vi "mes~产品出站.vi"(8 "error in (no error)":errorcluster caption="错误输入（无错误）", 11 "测试结果":string caption="测试结果:") -> (0 "error out":errorcluster caption="错误输出", 2 "出站成功":bool)   [LabVIEW 2015]
uses:
  ctl/SendOutStationCommon.ctl
  ctl/ReceiveOutStationCommon.ctl
  Global.vi
panel:
  in  "Headers":string[][](array[string])=[["Content-Type", "text/xml;charset=UTF-8"], ["SOAPAction", "\"http://tempuri.org/IOutStationServiceImpl/outStationService\""], ["Connection", "Keep-Alive"], ["User-Agent", "Apache-HttpClient/4.1.1 (java 1.5)"]]
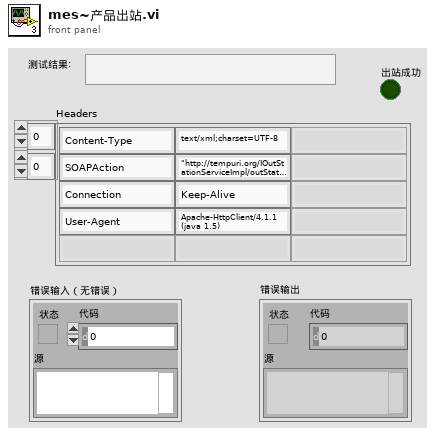
[diagram p1: front panel]
types:
  T1 = typedef "SendOutStationCommon.ctl" = cluster{"#attributes":cluster{"xmlns:soapenv":string, "xmlns:tem":string, "xmlns:cal":string}, "soapenv:Header":string, "soapenv:Body":cluster{"tem:outStationService":cluster{"tem:model":cluster{"cal:completeQty":string, "cal:equipNum":string, "cal:identiftyList":cluster{"cal:OutStationV01":cluster{"cal:identification":string, "cal:qualityStatus":string}[]}, "cal:productType":string, "cal:siteCode":string, "cal:testOrderNum":string}}}}
  T2 = cluster{"接口地址(URL)":string, "设备编号(equipNum)":string, "站点名称(siteCode)":string, "生产类型(productType)":string, "试验单号(testOrderNum)":string}
  T3 = typedef "ReceiveOutStationCommon.ctl" = cluster{"#attributes":cluster{"xmlns:s":string}, "s:Body":cluster{"outStationServiceResponse":cluster{"#attributes":cluster{"xmlns":string}, "outStationServiceResult":cluster{"#attributes":cluster{"xmlns:a":string, "xmlns:i":string}, "a:ErrorCode":string, "a:ErrorMessage":string, "a:Success":string}}}}
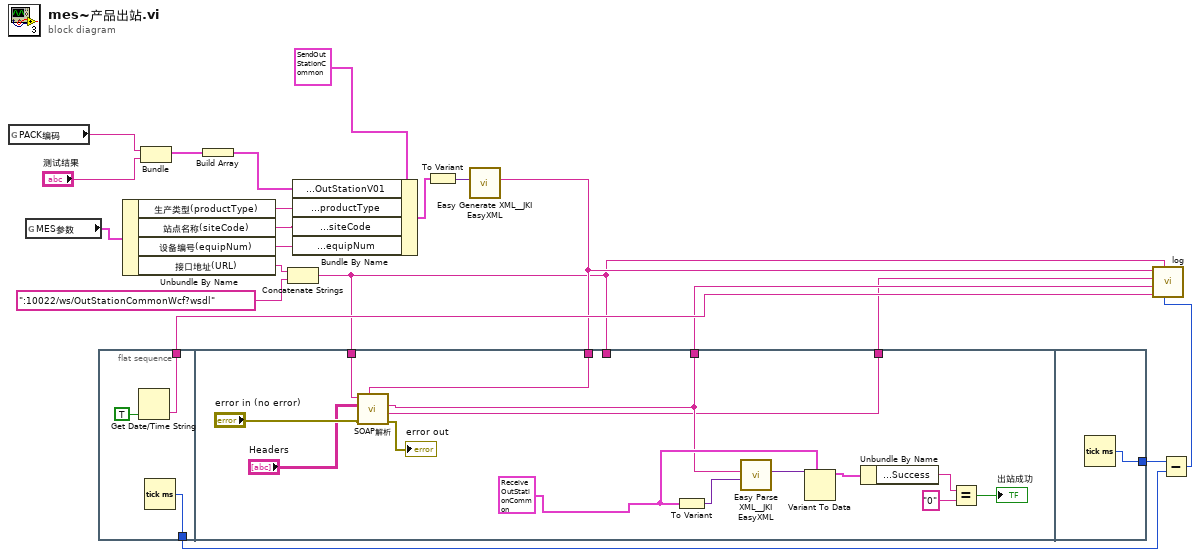
[diagram p0: block diagram]
diagram:
  n1 = global read "Global.vi" "PACK编码"() -> (w13:string)
  n2 = global read "Global.vi" "MES参数"() -> (w17:T2)
  n3 = flat-sequence {
    tunnel: [w23] -> w8
    tunnel: [w22] -> w7
    tunnel: w2 -> [_]
    tunnel: w5 -> [w28]
    tunnel: [w27] -> w4
    tunnel: w2 -> [w29]
    tunnel: [w25] -> w1
    tunnel: [w39] -> w9
    frame #0 {
      n4 = Get Date/Time String(want seconds? (F)=TRUE ("需要秒？(F)")) -> (time string=w22:string)  [unwired: 2 in, 1 out]
      n5 = Tick Count (ms)() -> (millisecond timer value=w23:u32)
    }
    frame #1 {
      w32 = T3 {"#attributes"={"xmlns:s"="http://schemas.xmlsoap.org/soap/envelope/"}, "s:Body"={"outStationServiceResponse"={"#attributes"={"xmlns"="http://tempuri.org/"}, "outStationServiceResult"={"#attributes"={"xmlns:a"="http://schemas.datacontract.org/2004/07/EdgeUtility", "xmlns:i"="http://www.w3.org/2001/XMLSchema-instance"}, "a:ErrorCode"="", "a:ErrorMessage"="", "a:Success"=""}}}} ("s:Envelope")
      n6 = call "SOAP解析.vi"("DATA"=w28, "错误输入（无错误）"="error in (no error)", "Headers"="Headers", "URL"=w29) -> ("错误输出"=→"error out":errorcluster, "headers"=w25:string, "body"=w27:string)  [unwired: 5 in]
      n7 = To Variant(anything=w32) -> (Variant=w38:variant)
      n8 = call <vilib>:"Easy Parse XML__JKI EasyXML.vi"("LabVIEW Data (Type)"=w38, "XML String"=w27) -> ("LabVIEW Data"=w37:variant)  [unwired: 8 in, 1 out]
      n9 = Variant To Data(type=w32, Variant=w37) -> (data=w36:T3)  [unwired: 1 in, 1 out]
      n10 = Unbundle By Name(w36) -> ("s:Body.outStationServiceResponse.outStationServiceResult.a:Success"=w35:string)
      n11 = Equal?(x=w35, y="0") -> (x = y?=→"出站成功":bool)
    }
    frame #2 {
      n12 = Tick Count (ms)() -> (millisecond timer value=w39:u32)
    }
  }
  n13 = Unbundle By Name(w17) -> ("生产类型(productType)"=w14:string, "站点名称(siteCode)"=w18:string, "设备编号(equipNum)"=w19:string, "接口地址(URL)"=w16:string)
  n14 = Bundle("PACK编码"=w13, "测试结果"="测试结果") -> (w11:cluster{"PACK编码":string, "测试结果":string})  [unwired: 1 in]
  n15 = Build Array(w11) -> (w10:cluster{"PACK编码":string, "测试结果":string}[])
  n16 = Concatenate Strings(w16, ":10022/ws/OutStationCommonWcf?wsdl") -> (w2:string)
  n17 = Bundle By Name(cluster=T1 {"#attributes"={"xmlns:soapenv"="http://schemas.xmlsoap.org/soap/envelope/", "xmlns:tem"="http://tempuri.org/", "xmlns:cal"="http://schemas.datacontract.org/2004/07/CalbOutStationCommonService"}, "soapenv:Header"="", "soapenv:Body"={"tem:outStationService"={"tem:model"={"cal:completeQty"="", "cal:equipNum"="", "cal:identiftyList"={"cal:OutStationV01"=[]}, "cal:productType"="", "cal:siteCode"="", "cal:testOrderNum"=""}}}} ("soapenv:Envelope"), "soapenv:Body.tem:outStationService.tem:model.cal:identiftyList.cal:OutStationV01"=w10, "soapenv:Body.tem:outStationService.tem:model.cal:productType"=w14, "soapenv:Body.tem:outStationService.tem:model.cal:siteCode"=w18, "soapenv:Body.tem:outStationService.tem:model.cal:equipNum"=w19) -> (w21:T1)
  n18 = To Variant(anything=w21) -> (Variant=w20:variant)
  n19 = call <vilib>:"Easy Generate XML__JKI EasyXML.vi"("LabVIEW Data"=w20) -> ("XML String"=w5:string)  [unwired: 9 in, 1 out]
  n20 = Subtract(x=w9, y=w8) -> (x-y=w6:u32)
  n21 = call "log.vi"("接口耗时"=w6, "URL"=w2, "StartTime"=w7, "响应报文"=w4, "header"=w1, "发送报文"=w5) -> ()  [unwired: 6 in]
